vi "ROSmsg_GetDataTypes.vi"(8 "error in":errorcluster, 11 "Msg Path":path) -> (0 "error out":errorcluster, 1 "Data Types":string[](array[string]), 2 "package path":path, 3 "Data Labels":string[](array[string]), 5 "msg name":string)   [LabVIEW 2012]
doc: "Scan through a message and pull out all the data types that will be contained in the message. If a data type shows up twice in the message, it will be listed twice in the array. This is to ensure that all the data is parsed and listed in the right order."
panel:
  out "Comments":string[](array[string])
  out "msg def":string
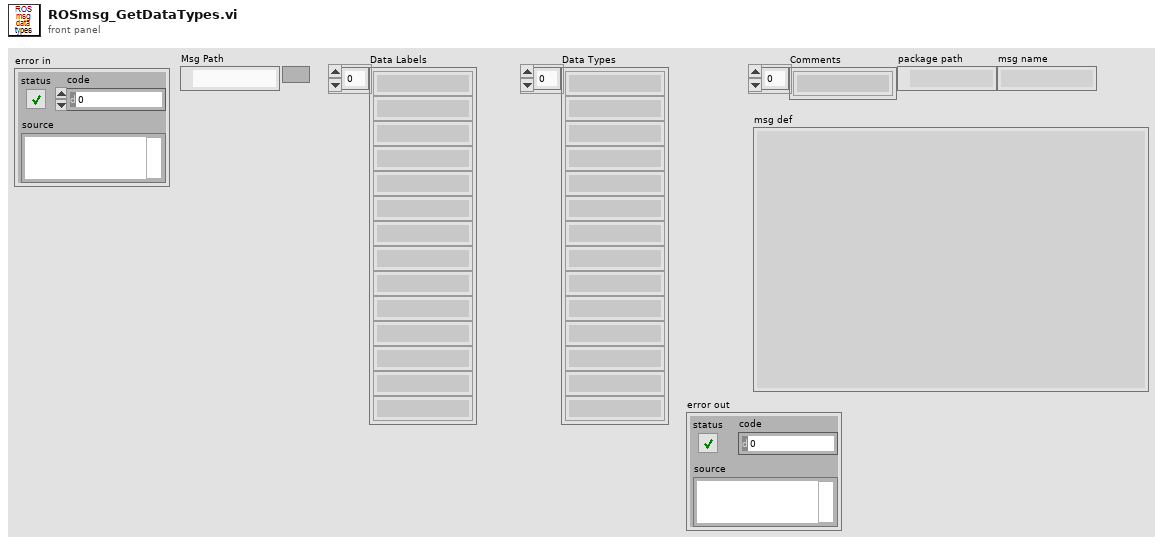
[diagram p1: front panel]
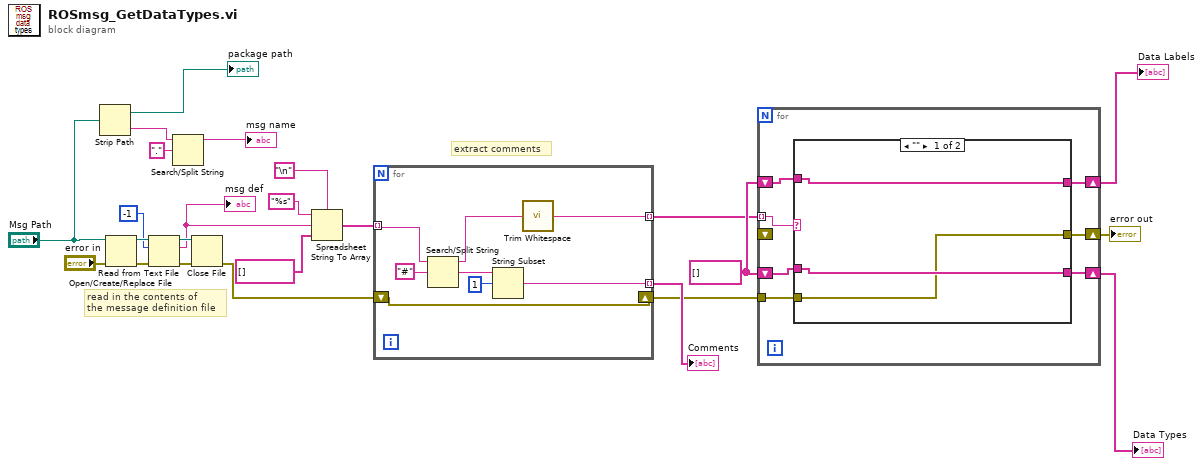
[diagram p0: block diagram]
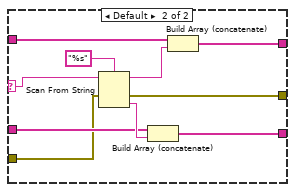
[diagram p2: hidden frame]
diagram:
  w23 = string[] []
  # "extract comments"
  # "read in the contents of\nthe message definition file"
  n1 = Strip Path(path="Msg Path") -> (stripped path=→"package path":path, name=w3:string)
  n2 = Open/Create/Replace File(file path (use dialog)="Msg Path", error in="error in") -> (refnum out=w18:refnum<file>, error out=w17:errorcluster)  [unwired: 4 in, 1 out]
  n3 = Read from Text File(file (use dialog)=w18, count=-1, error in=w17) -> (refnum out=w15:refnum<file>, text=w14:string, error out=w16:errorcluster)  [unwired: 1 in, 1 out]
  "msg def" <- w14
  n4 = Search/Split String(string=w3, search string/char (-)=".") -> (substring before match=→"msg name":string)  [unwired: 1 in, 2 out]
  n5 = Close File(refnum=w15, error in=w16) -> (error out=w8:errorcluster)  [unwired: 1 out]
  n6 = Spreadsheet String To Array(delimiter (Tab)="\n", format string="%s", spreadsheet string=w14, array type (2D Dbl)=string[] []) -> (array=w19:string[])
  n7 = for {
    tunnel: w19 -> [w29] mode=indexing
    tunnel: [w27] -> w21 mode=indexing
    tunnel: [w26] -> w20 mode=indexing
    shift-right: [w25] -> w7
    shift-left: w8 -> [w25]
    n8 = Search/Split String(string=w29, search string/char (-)="#") -> (substring before match=w28:string, match + rest of string=w31:string)  [unwired: 1 in, 1 out]
    n9 = String Subset(string=w31, offset (0)=1) -> (substring=w26:string)  [unwired: 1 in]
    n10 = call <vilib>:"Trim Whitespace.vi"("string"=w28) -> ("trimmed string"=w27:string)  [unwired: 1 in]
  }
  "Comments" <- w20
  n11 = for {
    tunnel: w21 -> [w39] mode=indexing
    shift-right: [w37] -> w22
    shift-left: w23 -> [w38]
    shift-right: [w36] -> w24
    shift-left: w23 -> [w35]
    shift-right: [w34] -> w6
    shift-left: _ -> [_]
    tunnel: w7 -> [w33]
    n12 = case shown="\"\"" w39 {
      selector: w39 -> [_ w51]
      tunnel: w38 -> [w42 w49]
      tunnel: [w42 w48] -> w37
      tunnel: [w41 w46] -> w36
      tunnel: w35 -> [w41 w45]
      tunnel: [w40 w44] -> w34
      tunnel: w33 -> [w40 w43]
      frame "" {
      }
      frame Default {
        n13 = Scan From String(format string="%s", input string=w51, error in=w43) -> (remaining string=w47:string, error out=w44:errorcluster, output 1=w50:string)  [unwired: 2 in, 1 out]
        n14 = Build Array (concatenate)(w49, w50) -> (w48:string[])
        n15 = Build Array (concatenate)(w45, w47) -> (w46:string[])
      }
    }
  }
  "Data Labels" <- w24
  "Data Types" <- w22
  "error out" <- w6
